vi "Filter Calc.vi"(8 "error in (no error)":errorcluster, 9 "Node Data":T2, 10 "Node Path (parent, child)":string[](array[string]), 11 "Filter Demo in":refnum<class "Filter Demo.lvclass">) -> (0 "error out":errorcluster, 1 "Keep options":T1, 2 "Keep node?":bool, 3 "Filter Demo out":refnum<class "Filter Demo.lvclass">)   [LabVIEW 2020, in "BlueTreeMapExamples OpenSource.lvlib" / "Filter Demo.lvclass"]
uses:
  Filter Demo.lvclass
  Typedefs/Tree Node Data.ctl
  Typedefs/Attribute Map.ctl
  Typedefs/Filter calc option.ctl
  Filter Demo.lvclass/Filter Demo.ctl
  Blue Tree Map OpenSource.lvlib
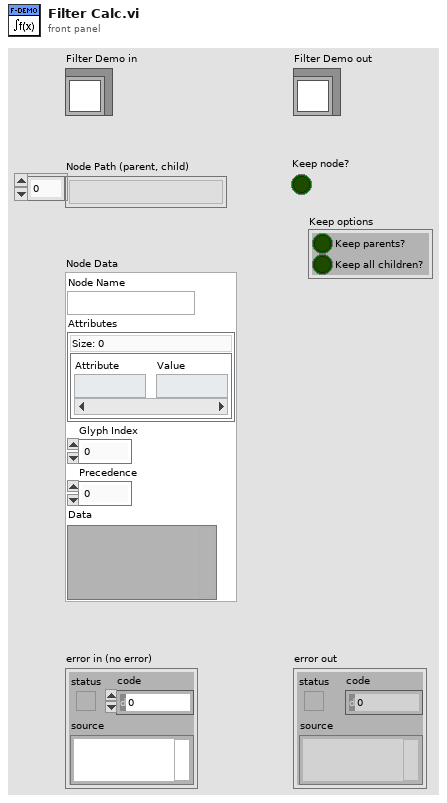
[diagram p1: front panel]
types:
  T1 = typedef "Blue Tree Map OpenSource.lvlib/Filter calc option.ctl" = cluster{"Keep parents?":bool, "Keep all children?":bool}
  T2 = typedef "Blue Tree Map OpenSource.lvlib/Tree Node Data.ctl" = cluster{"Node Name":string, "Attributes":T3, "Glyph Index":i32, "Precedence":i32, "Data":variant}
  T3 = typedef "Blue Tree Map OpenSource.lvlib/Attribute Map.ctl" = map{string, string}
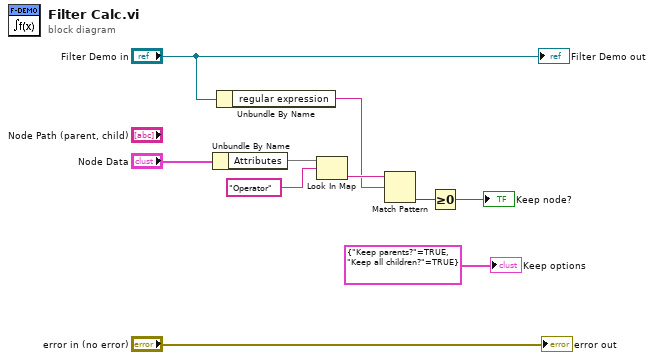
[diagram p0: block diagram]
diagram:
  n1 = Unbundle By Name("Node Data") -> ("Attributes"=w8:T3)
  n2 = Unbundle By Name("Filter Demo in") -> ("regular expression"=w5:string)
  n3 = Look In Map(map=w8, key="Operator") -> (value=w6:string)  [unwired: 1 in, 1 out]
  n4 = Match Pattern(string=w6, regular expression=w5) -> (offset past match=w3:i32)  [unwired: 1 in, 3 out]
  n5 = Greater Or Equal To 0?(x=w3) -> (x >= 0?=→"Keep node?":bool)
  "error out" <- "error in (no error)"
  "Filter Demo out" <- "Filter Demo in"
  "Keep options" <- T1 {"Keep parents?"=TRUE, "Keep all children?"=TRUE} ("Keep options")
